vi "Auto Play Path.vi"(8 "Operation":T2, 9 "Auto Data":T13, 10 "Motors":T3={"Drive Motors (NEO)"={"Left Front"={"DeviceStatus"={"status"=FALSE, "code"=0, "source"=""}, "Type"=enum."PWM", "PWM"={"PWM Channel"=enum."PWM 0", "DeadBand"={"Name"="", "maxPositivePwm"=0, "minPositivePwm"=0, "centerPwm"=0, "maxNegativePwm"=0, "minNegativePwm"=0, "angularRange"=0}}, "CAN"={"Device Number"=0, "SetOutput VI Ref"=variant, "GetOutput VI Ref"=variant, "Enable VI Ref"=variant, "Disable VI Ref"=variant, "Data"=variant}, "Invert"=FALSE, "DIO PWM"={"PWM \"Enable\" Channel"=enum."PWM 0", "DIOChannel"=enum."DIO 0", "PWM Rate"=0.0}}, "Left Back"={"DeviceStatus"={"status"=FALSE, "code"=0, "source"=""}, "Type"=enum."PWM", "PWM"={"PWM Channel"=enum."PWM 0", "DeadBand"={"Name"="", "maxPositivePwm"=0, "minPositivePwm"=0, "centerPwm"=0, "maxNegativePwm"=0, "minNegativePwm"=0, "angularRange"=0}}, "CAN"={"Device Number"=0, "SetOutput VI Ref"=variant, "GetOutput VI Ref"=variant, "Enable VI Ref"=variant, "Disable VI Ref"=variant, "Data"=variant}, "Invert"=FALSE, "DIO PWM"={"PWM \"Enable\" Channel"=enum."PWM 0", "DIOChannel"=enum."DIO 0", "PWM Rate"=0.0}}, "Right Front"={"DeviceStatus"={"status"=FALSE, "code"=0, "source"=""}, "Type"=enum."PWM", "PWM"={"PWM Channel"=enum."PWM 0", "DeadBand"={"Name"="", "maxPositivePwm"=0, "minPositivePwm"=0, "centerPwm"=0, "maxNegativePwm"=0, "minNegativePwm"=0, "angularRange"=0}}, "CAN"={"Device Number"=0, "SetOutput VI Ref"=variant, "GetOutput VI Ref"=variant, "Enable VI Ref"=variant, "Disable VI Ref"=variant, "Data"=variant}, "Invert"=FALSE, "DIO PWM"={"PWM \"Enable\" Channel"=enum."PWM 0", "DIOChannel"=enum."DIO 0", "PWM Rate"=0.0}}, "Right Back"={"DeviceStatus"={"status"=FALSE, "code"=0, "source"=""}, "Type"=enum."PWM", "PWM"={"PWM Channel"=enum."PWM 0", "DeadBand"={"Name"="", "maxPositivePwm"=0, "minPositivePwm"=0, "centerPwm"=0, "maxNegativePwm"=0, "minNegativePwm"=0, "angularRange"=0}}, "CAN"={"Device Number"=0, "SetOutput VI Ref"=variant, "GetOutput VI Ref"=variant, "Enable VI Ref"=variant, "Disable VI Ref"=variant, "Data"=variant}, "Invert"=FALSE, "DIO PWM"={"PWM \"Enable\" Channel"=enum."PWM 0", "DIOChannel"=enum."DIO 0", "PWM Rate"=0.0}}}, "Steer Motors (NEO)"={"Left Front"={"DeviceStatus"={"status"=FALSE, "code"=0, "source"=""}, "Type"=enum."PWM", "PWM"={"PWM Channel"=enum."PWM 0", "DeadBand"={"Name"="", "maxPositivePwm"=0, "minPositivePwm"=0, "centerPwm"=0, "maxNegativePwm"=0, "minNegativePwm"=0, "angularRange"=0}}, "CAN"={"Device Number"=0, "SetOutput VI Ref"=variant, "GetOutput VI Ref"=variant, "Enable VI Ref"=variant, "Disable VI Ref"=variant, "Data"=variant}, "Invert"=FALSE, "DIO PWM"={"PWM \"Enable\" Channel"=enum."PWM 0", "DIOChannel"=enum."DIO 0", "PWM Rate"=0.0}}, "Left Back"={"DeviceStatus"={"status"=FALSE, "code"=0, "source"=""}, "Type"=enum."PWM", "PWM"={"PWM Channel"=enum."PWM 0", "DeadBand"={"Name"="", "maxPositivePwm"=0, "minPositivePwm"=0, "centerPwm"=0, "maxNegativePwm"=0, "minNegativePwm"=0, "angularRange"=0}}, "CAN"={"Device Number"=0, "SetOutput VI Ref"=variant, "GetOutput VI Ref"=variant, "Enable VI Ref"=variant, "Disable VI Ref"=variant, "Data"=variant}, "Invert"=FALSE, "DIO PWM"={"PWM \"Enable\" Channel"=enum."PWM 0", "DIOChannel"=enum."DIO 0", "PWM Rate"=0.0}}, "Right Front"={"DeviceStatus"={"status"=FALSE, "code"=0, "source"=""}, "Type"=enum."PWM", "PWM"={"PWM Channel"=enum."PWM 0", "DeadBand"={"Name"="", "maxPositivePwm"=0, "minPositivePwm"=0, "centerPwm"=0, "maxNegativePwm"=0, "minNegativePwm"=0, "angularRange"=0}}, "CAN"={"Device Number"=0, "SetOutput VI Ref"=variant, "GetOutput VI Ref"=variant, "Enable VI Ref"=variant, "Disable VI Ref"=variant, "Data"=variant}, "Invert"=FALSE, "DIO PWM"={"PWM \"Enable\" Channel"=enum."PWM 0", "DIOChannel"=enum."DIO 0", "PWM Rate"=0.0}}, "Right Back"={"DeviceStatus"={"status"=FALSE, "code"=0, "source"=""}, "Type"=enum."PWM", "PWM"={"PWM Channel"=enum."PWM 0", "DeadBand"={"Name"="", "maxPositivePwm"=0, "minPositivePwm"=0, "centerPwm"=0, "maxNegativePwm"=0, "minNegativePwm"=0, "angularRange"=0}}, "CAN"={"Device Number"=0, "SetOutput VI Ref"=variant, "GetOutput VI Ref"=variant, "Enable VI Ref"=variant, "Disable VI Ref"=variant, "Data"=variant}, "Invert"=FALSE, "DIO PWM"={"PWM \"Enable\" Channel"=enum."PWM 0", "DIOChannel"=enum."DIO 0", "PWM Rate"=0.0}}}, "PigeonIMUDevRef"={"DeviceStatus"={"status"=FALSE, "code"=0, "source"=""}, "Device Number"=0, "Type"=352321536, "Device ID"=0, "Handle"=0, "UsageFrame"=0, "Library Path"=path ""}, "Radii (ft)"={"Left Front Position"=[], "Left Back Position"=[], "Right Front Position"=[], "Right Back Position"=[]}} {"PigeonIMUDevRef"."Type" items=["CAN"=352321536, "TalonSRX"=33554432]; "Radii (ft)"."Right Back Position" format="%.2f"; "Radii (ft)"."Right Front Position" format="%.2f"; "Radii (ft)"."Left Back Position" format="%.2f"; "Radii (ft)"."Left Front Position" format="%.2f"}) -> (0 "Auto Done?":bool, 2 "BotPose":cluster{"Numeric":dbl, "Numeric":dbl}[](array[cluster]), 3 "Bordeaux Pos":cluster{dbl, dbl}[](array[cluster]))   [LabVIEW 2025]
uses:
  swerve-template/Type Definitions/Data/Robot Velocities.ctl
  swerve-template/Type Definitions/Hardware/Swerve Drives/(NEO-NEO-ThroughBore-Pigeon2) Swerve.ctl
  swerve-template/Type Definitions/Hardware/4 Motor Sets/(NEO & NEO 550) 4 Motor Set.ctl
  <vilib>/Rock Robotics/WPI/MotorControl/WPI_MotorControlDeviceRef.ctl
  <vilib>/Rock Robotics/WPI/MotorControl/WPI_MotorControlType.ctl
  <vilib>/Rock Robotics/SystemInterfaces/DIO/FPGA_DIOPWMChannel.ctl
  <vilib>/Rock Robotics/WPI/PWM/WPI_PWMDeadband.ctl
  <vilib>/Rock Robotics/SystemInterfaces/DIO/FPGA_DIOChannel.ctl
  <vilib>/Rock Robotics/WPI/ThirdParty/Phoenix-LabVIEW/Pigeon IMU/CTRE_PigeonIMU_DeviceRef.ctl
  <vilib>/Rock Robotics/WPI/ThirdParty/Phoenix-LabVIEW/Pigeon IMU/CTRE_PigeonIMU_ConnectionType.ctl
  swerve-template/Type Definitions/Data/Pod Positions.ctl
  Implementation/Drive Operations.ctl
  <vilib>/Platform/TimedLoop/XDataNode/timing_clust.ctl
  <vilib>/Platform/TimedLoop/XDataNode/nitl_modes.ctl
  <vilib>/Platform/TimedLoop/XDataNode/wakeup.ctl
  <vilib>/Rock Robotics/WPI/ThirdParty/REV Robotics/REVLib/Typedef/Spark MAX Control Type.ctl
  <vilib>/Rock Robotics/WPI/DriverStation/WPI_DriverStationRobotMode2.ctl
  Framework/Robot Global Data.vi
  <vilib>/Platform/TimedLoop/XDataNode/XDataNode.xnode
  <vilib>/Platform/TimedLoop/XDataNode/XDNodeRunTimeDep.lvlib
panel:
  out "Array":T1[](array[typedef])
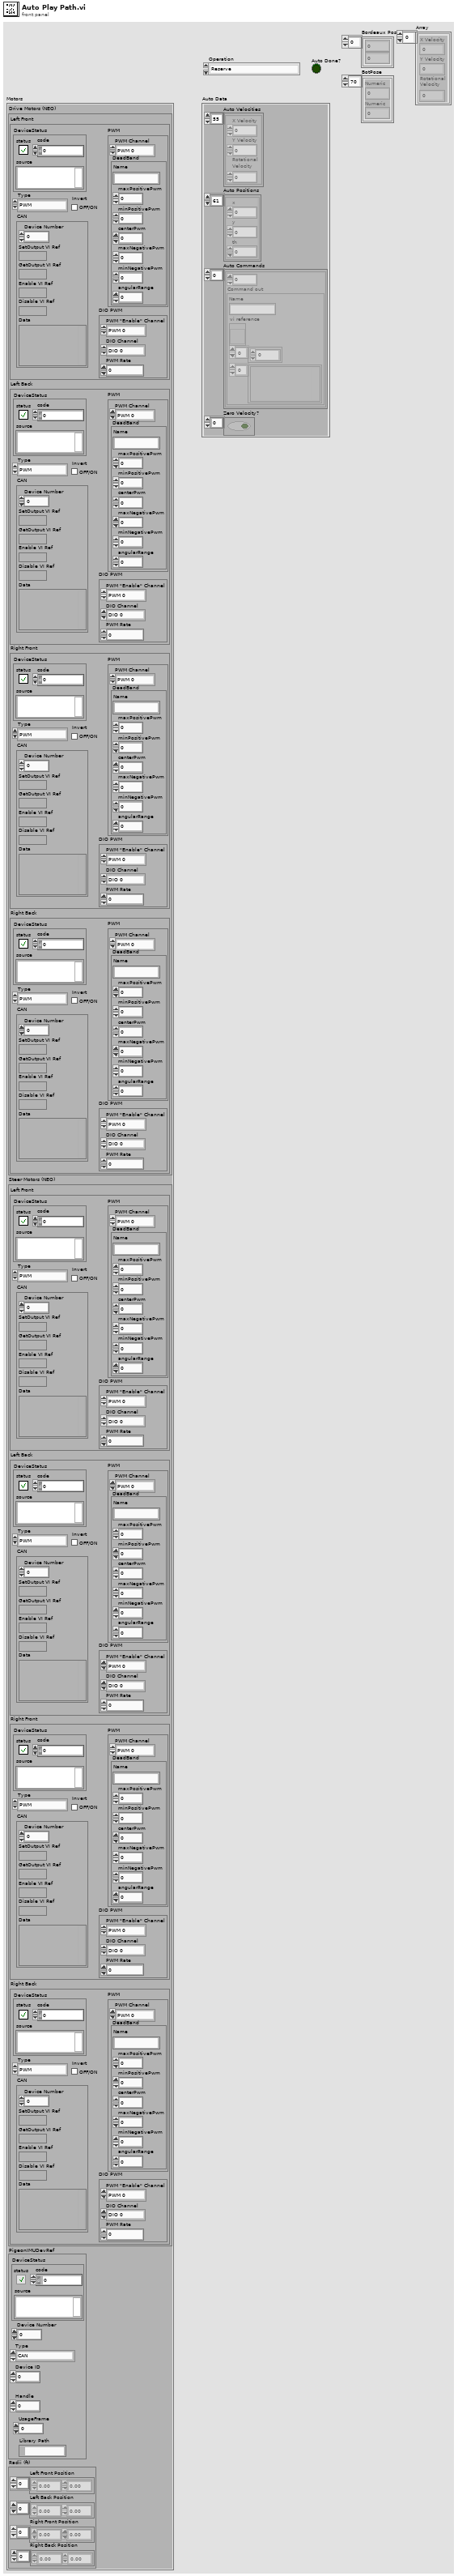
[diagram p1: front panel]
types:
  T1 = typedef "Robot Velocities.ctl" = cluster{"X Velocity":dbl, "Y Velocity":dbl, "Rotational \nVelocity":dbl}
  T2 = typedef "Drive Operations.ctl" = enum16{"Reserve", "Read Current", "Immediate", "Calibrate", "Auto", "Auto Pickup"}
  T3 = typedef "(NEO-NEO-ThroughBore-Pigeon2) Swerve.ctl" = cluster{"Drive Motors (NEO)":T4, "Steer Motors (NEO)":T4, "PigeonIMUDevRef":T10, "Radii (ft)":T12}
  T4 = typedef "(NEO & NEO 550) 4 Motor Set.ctl" = cluster{"Left Front":T5, "Left Back":T5, "Right Front":T5, "Right Back":T5}
  T5 = typedef "WPI_MotorControlDeviceRef.ctl" = cluster{"DeviceStatus":errorcluster, "Type":T6, "PWM":cluster{"PWM Channel":T7, "DeadBand":T8}, "CAN":cluster{"Device Number":u8, "SetOutput VI Ref":variant, "GetOutput VI Ref":variant, "Enable VI Ref":variant, "Disable VI Ref":variant, "Data":variant}, "Invert":bool, "DIO PWM":cluster{"PWM \"Enable\" Channel":T7, "DIOChannel":T9, "PWM Rate":dbl}}
  T6 = typedef "WPI_MotorControlType.ctl" = enum16{"PWM", "CAN", "DIO PWM"}
  T7 = typedef "FPGA_DIOPWMChannel.ctl" = enum8{"PWM 0", "PWM 1", "PWM 2", "PWM 3", "PWM 4", "PWM 5", "PWM 6", "PWM 7", "PWM 8", "PWM 9", "PWM MXP 0", "PWM MXP 1", "PWM MXP 2", "PWM MXP 3", "PWM MXP 4", "PWM MXP 5", "PWM MXP 6", "PWM MXP 7", "PWM MXP 8", "PWM MXP 9", "Invalid"}
  T8 = typedef "WPI_PWMDeadband.ctl" = cluster{"Name":string, "maxPositivePwm":i32, "minPositivePwm":i32, "centerPwm":i32, "maxNegativePwm":i32, "minNegativePwm":i32, "angularRange":u16}
  T9 = typedef "FPGA_DIOChannel.ctl" = enum8{"DIO 0", "DIO 1", "DIO 2", "DIO 3", "DIO 4", "DIO 5", "DIO 6", "DIO 7", "DIO 8", "DIO 9", "DIO MXP 0", "DIO MXP 1", "DIO MXP 2", "DIO MXP 3", "DIO MXP 4", "DIO MXP 5", "DIO MXP 6", "DIO MXP 7", "DIO MXP 8", "DIO MXP 9", "DIO MXP 10", "DIO MXP 11", "DIO MXP 12", "DIO MXP 13", "DIO MXP 14", "DIO MXP 15", "SPI Port CS1", "SPI Port CS2", "SPI Port CS3", "SPI Port MISO", "SPI Port MOSI", "Invalid"}
  T10 = typedef "CTRE_PigeonIMU_DeviceRef.ctl" = cluster{"DeviceStatus":errorcluster, "Device Number":u8, "Type":T11, "Device ID":u32, "Handle":u64, "UsageFrame":u32, "Library Path":path}
  T11 = typedef "CTRE_PigeonIMU_ConnectionType.ctl" = u32
  T12 = typedef "Pod Positions.ctl" = cluster{"Left Front Position":dbl[], "Left Back Position":dbl[], "Right Front Position":dbl[], "Right Back Position":dbl[]}
  T13 = cluster{"Auto Velocities":T1[], "Auto Positions":cluster{"x":dbl, "y":dbl, "th":dbl}[], "Auto Commands":cluster{dbl, "Command out":cluster{"Name":string, "vi reference":refnum<vi>, i32[], variant[]}}[], "Zero Velocity?":bool[]}
  T14 = cluster{"Time (s)":dbl, "Command out":cluster{"Name":string, "vi reference":refnum<vi>, i32[], variant[]}}
  T15 = typedef "Spark MAX Control Type.ctl" = enum16{"Percent VBus", "Voltage", "Velocity", "Position", "Smart Motion", "Current", "Smart Velocity", "MAXMotion Position", "MAXMotion Velocity"}
  T16 = cluster{"Left Front":dbl, "Left Back":dbl, "Right Front":dbl, "Right Back":dbl}
  T17 = cluster{dbl, "Command out":cluster{"Name":string, "vi reference":refnum<vi>, i32[], variant[]}}[]
  T18 = typedef "XDNodeRunTimeDep.lvlib/timing_clust.ctl" = cluster{"Expected End [f-1]":u64, "Actual End [f-1]":u64, "Finished Late? [f-1]":bool, "Expected End [i-1]":u64, "Actual End [i-1]":u64, "Finished Late? [i-1]":bool, "Expected Start [i]":u64, "Actual Start [i]":u64, "Expected Start [f]":u64, "Actual Start [f]":u64, "Source Name":string, "Structure Name":string, "Period":i64, "Deadline":i64, "Offset":i64, "Start":i64, "Priority":i32, "Timeout":i32, "Mode":T19, "Wakeup Reason":T20, "Error":errorcluster, "Source Type":string, "Secondary Source Type":string, "Global End Time":u64, "Global Start Time":u64, "Frame Duration":u64, "Iteration Duration":u64, "Assigned CPU":i32, "I/O Scan Engine Mode":u32}
  T19 = typedef "XDNodeRunTimeDep.lvlib/nitl_modes.ctl" = enum32{"No Change", "Process missed periods, maintain original phase", "Discard missed periods, maintain original phase", "Process missed periods, ignore original phase", "Discard missed periods, ignore original phase"}
  T20 = typedef "XDNodeRunTimeDep.lvlib/wakeup.ctl" = enum32{"Normal", "Aborted", "Asynchronous wakeup", "Timing source error", "Timed loop error", "Timeout"}
  T21 = typedef "WPI_DriverStationRobotMode2.ctl" = enum16{"Autonomous Disabled", "Autonomous Enabled", "Teleop Disabled", "Teleop Enabled", "Disconnected", "Finish", "Test Disabled", "Test Enabled", "Emergency Stopped"}
  T22 = typedef "Drive Conditions.ctl" = cluster{"Field Centric":bool, "Ball Pathing":bool, "Theta Align":bool, "Heavy PID":bool, "Align to Bump or Shoot":bool}
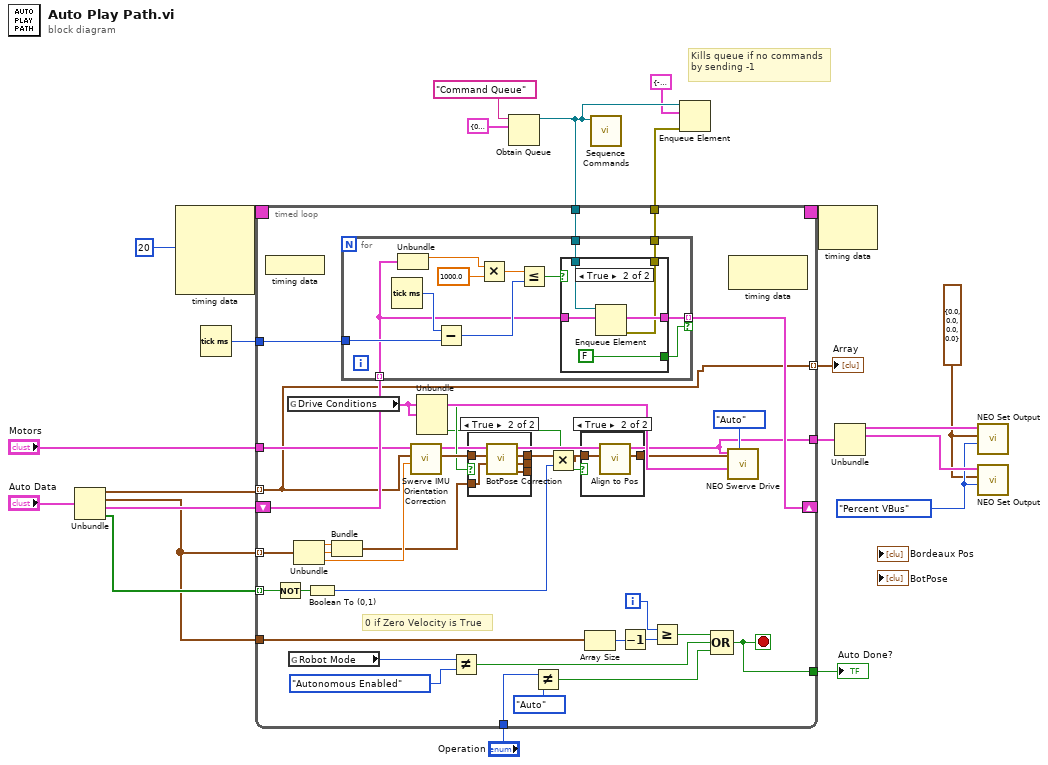
[diagram p0: block diagram]
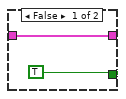
[diagram p4: hidden frame]
diagram:
  w11 = Spark_MAX_Control_Type."Percent VBus" ("Control Mode")
  w10 = T16 {"Left Front"=0.0, "Left Back"=0.0, "Right Front"=0.0, "Right Back"=0.0} ("Setpoints")
  # "Kills queue if no commands by sending -1"
  n1 = Unbundle("Auto Data") -> ("Auto Velocities"=w1:T1[], "Auto Positions"=w2:cluster{"x":dbl, "y":dbl, "th":dbl}[], "Auto Commands"=w20:T17, "Zero Velocity?"=w4:bool[])
  n2 = node-c288(i64 20 ("Period")) -> (w23:T18)  [unwired: 3 in]
  n3 = Tick Count (ms)() -> (millisecond timer value=w19:u32)
  n4 = Obtain Queue(name (unnamed)="Command Queue", element data type=T14 {"Time (s)"=0.0, "Command out"={"Name"="", "vi reference"=refnum, [], []}} ("element")) -> (queue out=w7:refnum<queue>)  [unwired: 3 in, 2 out]
  n5 = timed-loop {
    timing: w23 -> [_]
    timing-out: [_] -> w22
    tunnel: "Motors" -> [w29]
    tunnel: [w29] -> w9
    tunnel: w1 -> [w28] mode=indexing
    tunnel: w2 -> [w57] mode=indexing
    tunnel: w2 -> [w56]
    tunnel: w19 -> [w55]
    tunnel: w7 -> [w53]
    shift-right: [w51] -> _
    shift-left: w20 -> [w50]
    tunnel: w4 -> [w41] mode=indexing
    tunnel: [w44] -> w21
    tunnel: "Operation" -> [w40]
    tunnel: [w39] -> w6
    tunnel: [w28] -> w3 mode=indexing
    i -> [w58]
    stop <- w44 stop-if-true
    # "0 if Zero Velocity is True"
    n6 = node-c288() -> ()  [unwired: 1 in]
    n7 = Not(x=w41) -> (.not. x?=w47:bool)
    n8 = global read "Robot Global Data.vi" "Drive Conditions"() -> (w31:T22)
    n9 = global read "Robot Global Data.vi" "Robot Mode"() -> (w49:T21)
    n10 = Unbundle(w57) -> ("x"=w36:dbl, "y"=w35:dbl, "th"=w38:dbl)
    n11 = Boolean To (0,1)(Boolean=w47) -> (0, 1=w46:i16)
    n12 = Bundle("x"=w36, "y"=w35) -> (w34:cluster{"x":dbl, "y":dbl})  [unwired: 1 in]
    n13 = for {
      tunnel: w55 -> [w78]
      tunnel: w53 -> [w72]
      tunnel: w50 -> [w69] mode=indexing
      tunnel: [w71] -> w51 mode=indexing if=w70
      tunnel: [w68] -> w39
      n14 = Tick Count (ms)() -> (millisecond timer value=w79:u32)
      n15 = Unbundle(w69) -> (w77:dbl)  [unwired: 1 out]
      n16 = Subtract(x=w79, y=w78) -> (x-y=w74:u32)
      n17 = Multiply(x=w77, y=1000.0) -> (x*y=w75:dbl)
      n18 = Less Or Equal?(x=w75, y=w74) -> (x <= y?=w73:bool)
      n19 = case shown="True" w73 {
        tunnel: w72 -> [_ w85]
        tunnel: w69 -> [w80 w84]
        tunnel: [w80 w84] -> w71
        tunnel: [TRUE FALSE] -> w70
        tunnel: [_ w82] -> w68
        frame False {
        }
        frame True {
          n20 = Enqueue Element(queue=w85, element=w84) -> (error out=w82:errorcluster)  [unwired: 2 in, 2 out]
        }
      }
    }
    n21 = call "Swerve IMU Orientation Correction.vi"("Setpoint"=w38, "Robot Velocities In"=w28) -> ("Robot Velocities Out"=w37:T1)  [unwired: 9 in]
    n22 = Unbundle(w31) -> ("Ball Pathing"=w30:bool, "Align to Bump or Shoot"=w27:bool)  [unwired: 3 out]
    n23 = Not Equal?(x=w49, y=WPI_DriverStationRobotMode2."Autonomous Enabled") -> (x != y?=w45:bool)
    n24 = case shown="True" w30 {
      tunnel: w37 -> [w59 w64]
      tunnel: [w59 w63] -> w25
      tunnel: w34 -> [_ w62]
      tunnel: [_ w61] -> _
      tunnel: [_ w60] -> _
      frame False {
      }
      frame True {
        n25 = call "BotPose Correction.vi"("Pos In"=w62, "Robot Velocities In"=w64) -> ("BotPose"=w60:cluster{"Numeric":dbl, "Numeric":dbl}, "Bordeaux Pos"=w61:cluster{dbl, dbl}, "Robot Velocities Out"=w63:T1)  [unwired: 7 in]
      }
    }
    n26 = Not Equal?(x=w40, y=Drive_Operations."Auto") -> (x != y?=w43:bool)
    n27 = Multiply(x=w25, y=w46) -> (x*y=w24:T1)
    n28 = case shown="True" w27 {
      tunnel: [w65 w67] -> w26
      tunnel: w24 -> [w65 w66]
      frame False {
      }
      frame True {
        n29 = call "Align to Pos.vi"("Robot Velocities In"=w66) -> ("Robot Velocities Out"=w67:T1)  [unwired: 10 in]
      }
    }
    n30 = Array Size(array=w56) -> (size(s)=w32:i32)
    n31 = Decrement(x=w32) -> (x-1=w33:i32)
    n32 = Greater Or Equal?(x=w58, y=w33) -> (x >= y?=w54:bool)
    n33 = Compound Arithmetic op=OR(w54, w45, w43) -> (w44:bool)
    n34 = call "NEO Swerve Drive.vi"("Operation"=Drive_Operations."Auto", "Drive Conditions"=w31, "Robot Velocities"=w26, "Swerve Drive"=w29) -> ()  [unwired: 7 in, 1 out]
    n35 = node-c288() -> ()  [unwired: 1 in, 1 out]
  }
  "Auto Done?" <- w21
  "Array" <- w3
  n36 = call "Sequence Commands.vi"("queue in"=w7) -> ()  [unwired: 11 in]
  n37 = Enqueue Element(queue=w7, element=T14 {"Time (s)"=-1.0, "Command out"={"Name"="", "vi reference"=refnum, [], []}}, error in (no error)=w6) -> ()  [unwired: 1 in, 3 out]
  n38 = node-c288(w22) -> ()  [unwired: 1 out]
  n39 = Unbundle(w9) -> ("Drive Motors (NEO)"=w13:T4, "Steer Motors (NEO)"=w12:T4)  [unwired: 2 out]
  n40 = call "NEO Set Output.vi"("Control Mode"=w11, "Setpoints"=w10, "Motors"=w13) -> ()  [unwired: 9 in]
  n41 = call "NEO Set Output.vi"("Control Mode"=w11, "Setpoints"=w10, "Motors"=w12) -> ()  [unwired: 9 in]
